vi "Error Handler - Update Settings UI Loop.vi"(8 "Error In":errorcluster) -> (0 "Error Out":errorcluster)   [LabVIEW 2017]
uses:
  <vilib>/Utility/error.llb/DialogType.ctl
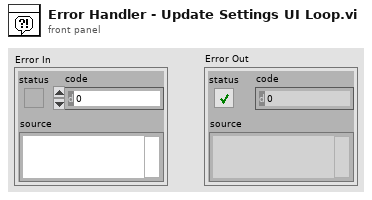
[diagram p1: front panel]
types:
  T1 = typedef "DialogType.ctl" = u16
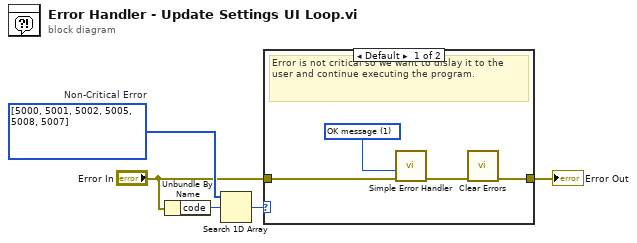
[diagram p0: block diagram]
diagram:
  w5 = i32[] [5000, 5001, 5002, 5005, 5008, 5007]  # Non-Critical Error
  n1 = Unbundle By Name("Error In") -> ("code"=w4:i32)
  n2 = Search 1D Array(1D array=w5, element=w4) -> (index of element=w3:i32)  [unwired: 1 in]
  n3 = case shown="Default" w3 {
    tunnel: "Error In" -> [w9 w10]
    tunnel: [w6 w10] -> w1
    frame Default {
      w8 = T1 1 items=["no dialog", "OK message", "continue or stop message", "OK message + warnings", "continue/stop + warnings"] ("type of dialog (OK msg:1)")
      # "Error is not critical so we want to dislay it to the user and continue executing the program."
      n4 = call <vilib>:"Simple Error Handler.vi"("type of dialog (OK msg:1)"=w8, "error in (no error)"=w9) -> ("error out"=w7:errorcluster)  [unwired: 3 in, 4 out]
      n5 = call <vilib>:"Clear Errors.vi"("error in (no error)"=w7) -> ("error out"=w6:errorcluster)  [unwired: 5 in, 1 out]
    }
    frame -1 {
      # "Dont ignore this error"
    }
  }
  "Error Out" <- w1
